vi "Set Class VIs Properties.vi"(7 "VI Options":T1, 8 "error in (no error)":errorcluster, 11 "class ref":refnum<vi>) -> (0 "error out":errorcluster, 3 "class vi refs":refnum<vi>[](array[refnum]))   [LabVIEW 2019, in "Build Automation.lvlib"]
uses:
  Build Automation.lvlib
  VI Options.ctl
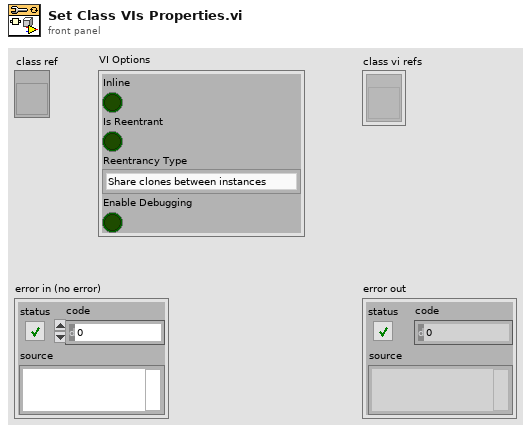
[diagram p1: front panel]
types:
  T1 = typedef "Build Automation.lvlib/VI Options.ctl" = cluster{"Inline":bool, "Is Reentrant":bool, "Reentrancy Type":enum16{"Share clones between instances", "Preallocate clone for each instance"}, "Enable Debugging":bool}
  T2 = enum16{"Share clones between instances", "Preallocate clone for each instance"}
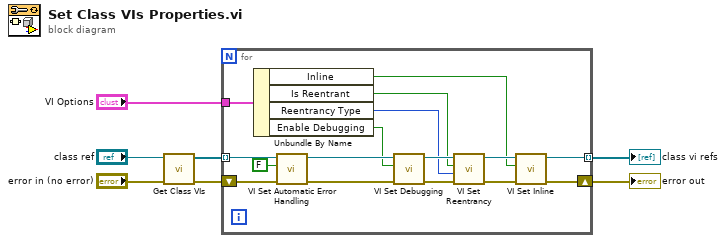
[diagram p0: block diagram]
diagram:
  n1 = call "Get Class VIs.vi"("error in (no error)"="error in (no error)", "class ref"="class ref") -> ("error out"=w4:errorcluster, "vi refs"=w5:refnum<vi>[])  [unwired: 8 in]
  n2 = for {
    tunnel: w5 -> [w22] mode=indexing
    shift-right: [w10] -> w2
    shift-left: w4 -> [w23]
    tunnel: "VI Options" -> [w18]
    tunnel: [w8] -> w1 mode=indexing
    n3 = Unbundle By Name(w18) -> ("Inline"=w9:bool, "Is Reentrant"=w13:bool, "Reentrancy Type"=w14:T2, "Enable Debugging"=w17:bool)
    n4 = call "VI Set Automatic Error Handling.vi"("error in (no error)"=w23, "Automatic Error Handling"=FALSE, "vi ref in"=w22) -> ("error out"=w19:errorcluster, "vi ref out"=w20:refnum<vi>)  [unwired: 7 in]
    n5 = call "VI Set Debugging.vi"("error in (no error)"=w19, "Allow Debugging"=w17, "vi ref in"=w20) -> ("error out"=w15:errorcluster, "vi ref out"=w16:refnum<vi>)  [unwired: 7 in]
    n6 = call "VI Set Reentrancy.vi"("error in (no error)"=w15, "Reentrancy Type (shared clone)"=w14, "Is Reentrant"=w13, "vi ref in"=w16) -> ("error out"=w11:errorcluster, "vi ref out"=w12:refnum<vi>)  [unwired: 6 in]
    n7 = call "VI Set Inline.vi"("error in (no error)"=w11, "Inline VI"=w9, "vi ref in"=w12) -> ("error out"=w10:errorcluster, "vi ref out"=w8:refnum<vi>)  [unwired: 7 in]
  }
  "error out" <- w2
  "class vi refs" <- w1
